vi "PFE GCD (CDB).vi"(6 "tolerance type":u16(ring) items=["Absolute", "Relative"], 8 "algorithm":u16(ring) items=["Euclidean", "Approximate GCD"], 9 "tolerance":dbl=1e-08, 10 "Q(x)":cdb[](array[numeric]) format="%#.6g", 11 "P(x)":cdb[](array[numeric]) format="%#.6g") -> (0 "error":i32, 3 "Greatest Common Divisor":cdb[](array[numeric]) format="%#.6g")   [LabVIEW 2017, in "NI_AALPro.lvlib"]
uses:
  NI_AALPro.lvlib
  Polynomial GCD Pair (CDB).vi
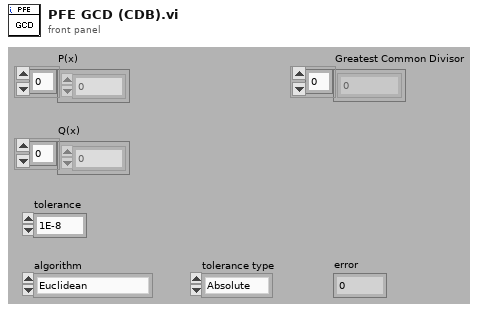
[diagram p1: front panel]
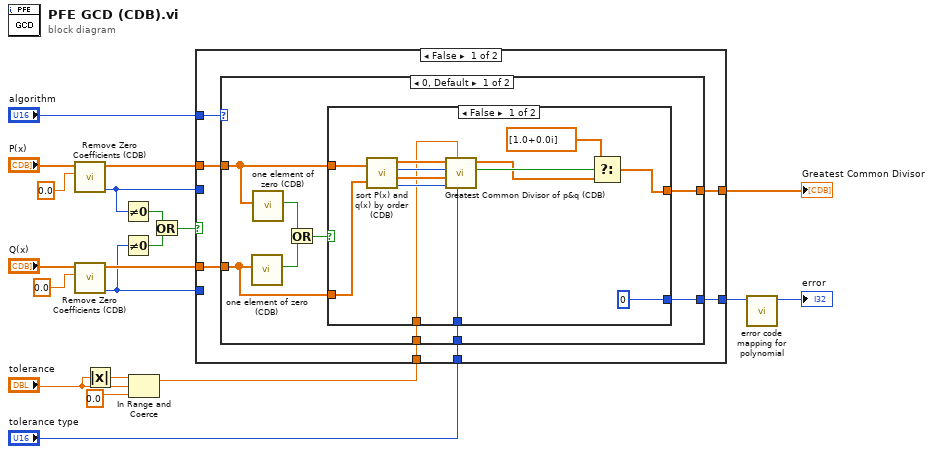
[diagram p0: block diagram]
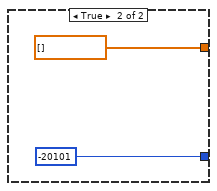
[diagram p2: hidden frame]
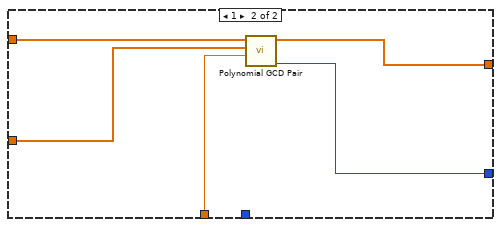
[diagram p3: hidden frame]
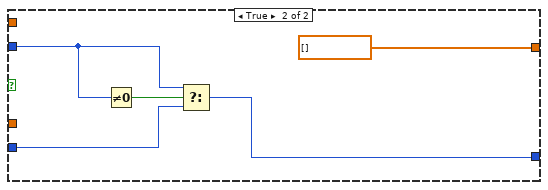
[diagram p4: hidden frame]
diagram:
  n1 = call "Remove Zero Coefficients (CDB).vi"("threshold"=0.0, "P(x) In"="P(x)") -> ("error"=w7:i32, "P(x) Out"=w17:cdb[])  [unwired: 7 in, 1 out]
  n2 = call "Remove Zero Coefficients (CDB).vi"("threshold"=0.0, "P(x) In"="Q(x)") -> ("error"=w6:i32, "P(x) Out"=w16:cdb[])  [unwired: 7 in, 1 out]
  n3 = Absolute Value(x="tolerance") -> (abs(x)=w13:dbl)
  n4 = Not Equal To 0?(x=w7) -> (x != 0?=w5:bool)
  n5 = Not Equal To 0?(x=w6) -> (x != 0?=w4:bool)
  n6 = In Range and Coerce(upper limit=w13, x="tolerance", lower limit=0.0) -> (coerced(x)=w10:dbl)  [unwired: 1 out]
  n7 = Or(x=w5, y=w4) -> (x .or. y?=w3:bool)
  n8 = case shown="False" w3 {
    tunnel: [w27 cdb[] [] ("CDB")] -> w20
    tunnel: w17 -> [w26 _]
    tunnel: w16 -> [w25 _]
    tunnel: [w24 w57] -> w9
    tunnel: w10 -> [w23 _]
    tunnel: w7 -> [_ w59]
    tunnel: w6 -> [_ w58]
    tunnel: "algorithm" -> [w22 _]
    tunnel: "tolerance type" -> [w21 _]
    frame False {
      n9 = case shown="0, Default" w22 {
        tunnel: [w36 w53] -> w27
        tunnel: w26 -> [w34 w56]
        tunnel: w25 -> [w31 w55]
        tunnel: [w30 w52] -> w24
        tunnel: w23 -> [w29 w54]
        tunnel: w21 -> [w28 _]
        frame 0, Default {
          n10 = call "one element of zero (CDB).vi"("Array in"=w31) -> ("equal [0]?"=w32:bool)  [unwired: 10 in]
          n11 = call "one element of zero (CDB).vi"("Array in"=w34) -> ("equal [0]?"=w33:bool)  [unwired: 10 in]
          n12 = Or(x=w33, y=w32) -> (x .or. y?=w35:bool)
          n13 = case shown="False" w35 {
            tunnel: w34 -> [w49 _]
            tunnel: w31 -> [w48 _]
            tunnel: [w47 cdb[] []] -> w36
            tunnel: [0 ("coef. of poly are all zero") -20101 ("coef. of poly are all zero")] -> w30
            tunnel: w29 -> [w42 _]
            tunnel: w28 -> [w41 _]
            frame False {
              n14 = call "sort P(x) and q(x) by order (CDB).vi"("p"=w49, "q"=w48) -> ("high order polynomial"=w46:cdb[], "high order"=w45:i32, "low order polynomial"=w44:cdb[], "low order"=w43:i32)
              n15 = call "Greatest Common Divisor of p&q (CDB).vi"("tolerance type"=w41, "tolerance"=w42, "order of q"=w43, "q"=w44, "order of p"=w45, "p"=w46) -> ("coprime?"=w40:bool, "greatest common factor"=w37:cdb[])  [unwired: 3 in, 1 out]
              n16 = Select(t=cdb[] [1.0+0.0i], s=w40, f=w37) -> (s? t:f=w47:cdb[])
            }
            frame True {
            }
          }
        }
        frame 1 {
          n17 = call-poly "Polynomial GCD Pair.vi"("tolerance"=w54, "Q(x)"=w55, "P(x)"=w56) -> ("error"=w52:i32, "Greatest Common Divisor"=w53:cdb[])  [unwired: 5 in, 2 out]
        }
      }
    }
    frame True {
      n18 = Not Equal To 0?(x=w59) -> (x != 0?=w60:bool)
      n19 = Select(t=w59, s=w60, f=w58) -> (s? t:f=w57:i32)
    }
  }
  "Greatest Common Divisor" <- w20
  n20 = call "error code mapping for polynomial.vi"("error in"=w9) -> ("error out"=→"error":i32)  [unwired: 10 in]
